vi "HEWH Assemble Test Sequence.vi"(8 "Error In":errorcluster, 11 "Cluster":T1 {"Time" format="%<%H:%M:%S>t"}) -> (0 "Error Out":errorcluster, 3 "String Test Seq":string[][](array[string]))   [LabVIEW 2016]
uses:
  Type Definitions/PRAT Test.ctl
  Utility/Save File/File Setup (Public)/Type Definition/Save File HEWH Heating Control Mode.ctl
  Draw Water Specific/Type Definitions/Terminate Draw Conditions.ctl
  Type Definitions/HEWH Start Conditions.ctl
  Draw Water Specific/Type Definitions/Check Special Condtions.ctl
  Draw Water Specific/Type Definitions/HEWH Special Condition Check.ctl
  Type Definitions/HEWH Draw Flag ENUM.ctl
  Utility/Save File/File Setup.lvlib
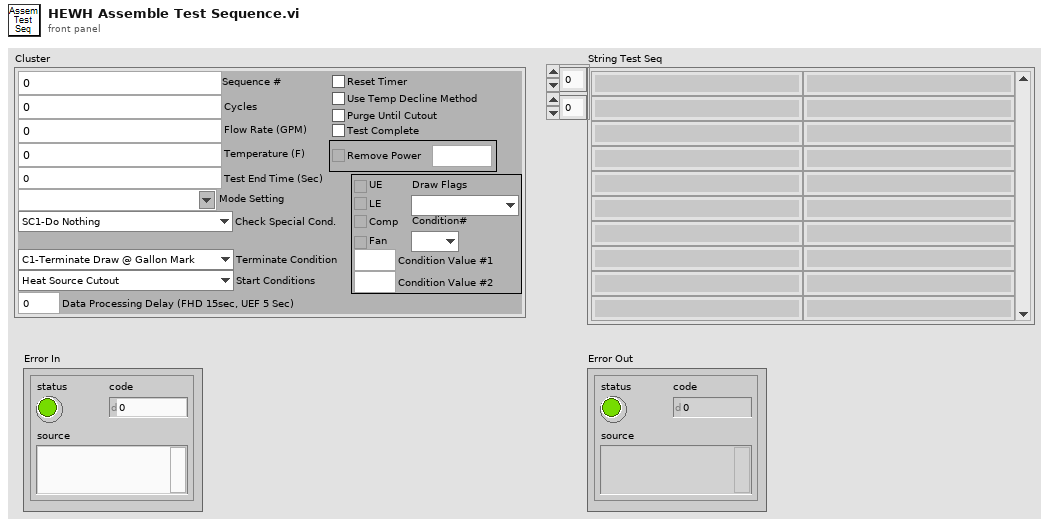
[diagram p1: front panel]
types:
  T1 = typedef "PRAT Test.ctl" = cluster{"Sequence #":dbl, "Cycles":i32, "Mode Setting":T2, "Flow Rate (GPM)":dbl, "Temperature (F)":dbl, "Reset Timer":bool, "Use Temp Decline Method":bool, "Terminate Condition":T3, "Condition Value #1":dbl, "UE":bool, "LE":bool, "Comp":bool, "Fan":bool, "Test End Time (Sec)":dbl, "Purge Until Cutout":bool, "Start Conditions":T4, "Condition Value #2":dbl, "Remove Power":bool, "Time":dbl, "Check Special Cond.":T5, "Condition#":T6, "Draw Flags":T7, "Data Processing Delay (FHD 15sec, UEF 5 Sec)":dbl, "Test Complete":bool}
  T2 = typedef "File Setup.lvlib/Save File HEWH Heating Control Mode.ctl" = string
  T3 = typedef "Terminate Draw Conditions.ctl" = enum16{"C1-Terminate Draw @ Gallon Mark", "C2-Special Last Draw (HU Test)", "C3-RTD Out <=", "C4-Mean Tank Temp <=", "C5-Decrease RTD Out (Deg F)", "C6-Time (Seconds)", "C7-Until Any Heat Source", "C8-Specific Heat Source", "C9-Do Nothing"}
  T4 = typedef "HEWH Start Conditions.ctl" = enum16{"Heat Source Cutout", "At Time (Seconds)", "Every X (Seconds)", "T2 >= X° Below Setpoint", "Seconds From Complete", "Wait for LE & Comp Cutout", "Wait for Comp Cutout", "Wait for LE Cutout", "Wait for UE Cutout"}
  T5 = typedef "Check Special Condtions.ctl" = enum16{"SC1-Do Nothing", "SC2-Check Heat Source (On-C2/Off-C1)", "SC3-Check Skip Condition", "SC4-Check Heat Source ON/Fail"}
  T6 = typedef "HEWH Special Condition Check.ctl" = enum16{"N/A", "C1", "C2", "Reset/Fail", "Skip Draw Sequence"}
  T7 = typedef "HEWH Draw Flag ENUM.ctl" = enum16{"N/A", "None(0)", "Sml(1)", "Med(2)", "SmlMed(3)", "Lrg(4)", "SmlLrg(5)", "MedLrg(6)", "SmlMedLrg(7)"}
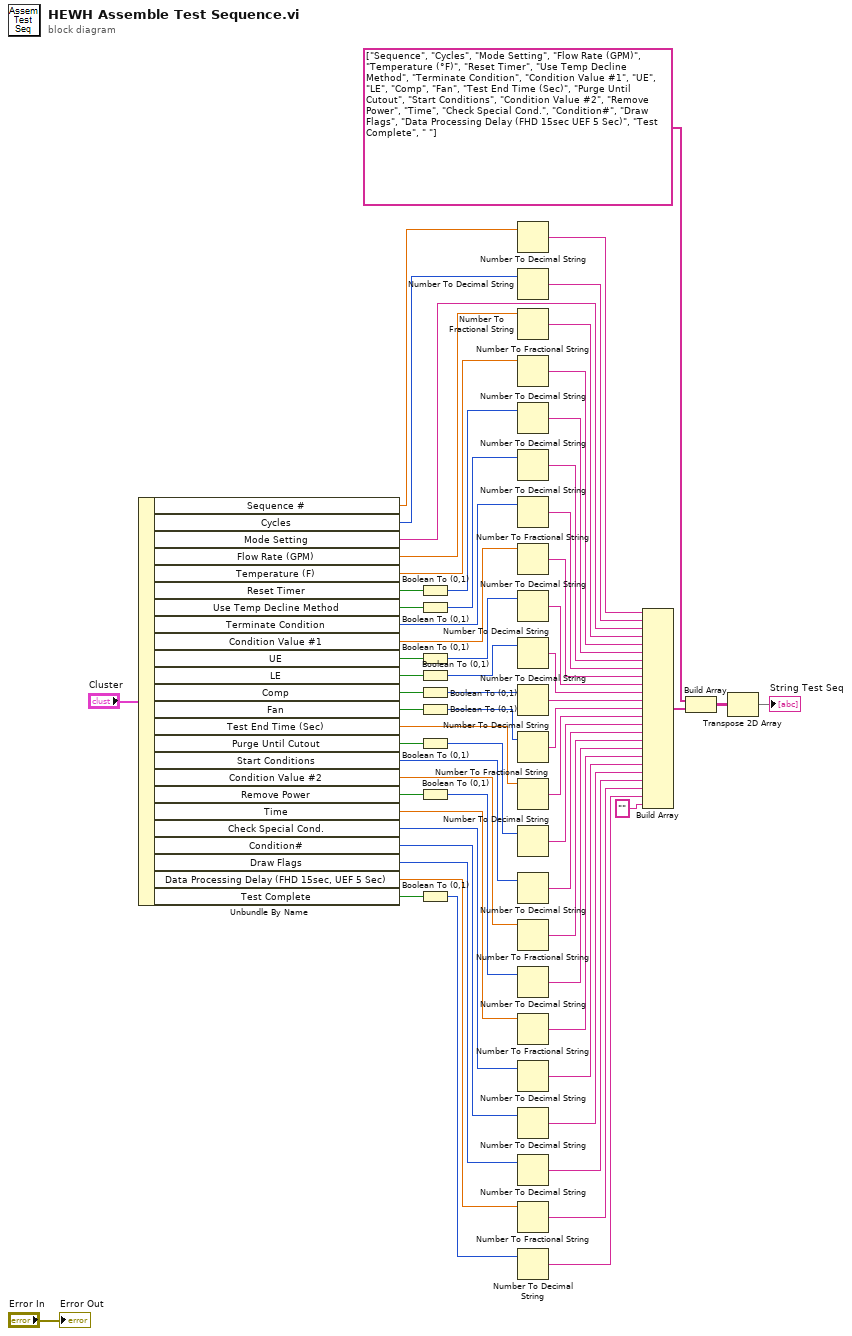
[diagram p0: block diagram]
diagram:
  n1 = Unbundle By Name("Cluster") -> ("Sequence #"=w3:dbl, "Cycles"=w9:i32, "Mode Setting"=w1:T2, "Flow Rate (GPM)"=w10:dbl, "Temperature (F)"=w11:dbl, "Reset Timer"=w12:bool, "Use Temp Decline Method"=w15:bool, "Terminate Condition"=w16:T3, "Condition Value #1"=w17:dbl, "UE"=w19:bool, "LE"=w21:bool, "Comp"=w23:bool, "Fan"=w25:bool, "Test End Time (Sec)"=w26:dbl, "Purge Until Cutout"=w28:bool, "Start Conditions"=w29:T4, "Condition Value #2"=w30:dbl, "Remove Power"=w32:bool, "Time"=w33:dbl, "Check Special Cond."=w34:T5, "Condition#"=w35:T6, "Draw Flags"=w36:T7, "Data Processing Delay (FHD 15sec, UEF 5 Sec)"=w37:dbl, "Test Complete"=w39:bool)
  n2 = Boolean To (0,1)(Boolean=w12) -> (0, 1=w13:i16)
  n3 = Boolean To (0,1)(Boolean=w15) -> (0, 1=w14:i16)
  n4 = Boolean To (0,1)(Boolean=w19) -> (0, 1=w18:i16)
  n5 = Boolean To (0,1)(Boolean=w21) -> (0, 1=w20:i16)
  n6 = Boolean To (0,1)(Boolean=w23) -> (0, 1=w22:i16)
  n7 = Boolean To (0,1)(Boolean=w25) -> (0, 1=w24:i16)
  n8 = Boolean To (0,1)(Boolean=w28) -> (0, 1=w27:i16)
  n9 = Boolean To (0,1)(Boolean=w32) -> (0, 1=w31:i16)
  n10 = Boolean To (0,1)(Boolean=w39) -> (0, 1=w38:i16)
  n11 = Number To Decimal String(number=w3) -> (decimal integer string=w2:string)  [unwired: 1 in]
  n12 = Number To Decimal String(number=w9) -> (decimal integer string=w40:string)  [unwired: 1 in]
  n13 = Number To Fractional String(number=w10) -> (F-format string=w41:string)  [unwired: 3 in]
  n14 = Number To Fractional String(number=w11) -> (F-format string=w42:string)  [unwired: 3 in]
  n15 = Number To Decimal String(number=w13) -> (decimal integer string=w43:string)  [unwired: 1 in]
  n16 = Number To Decimal String(number=w14) -> (decimal integer string=w44:string)  [unwired: 1 in]
  n17 = Number To Decimal String(number=w16) -> (decimal integer string=w45:string)  [unwired: 1 in]
  n18 = Number To Fractional String(number=w17) -> (F-format string=w46:string)  [unwired: 3 in]
  n19 = Number To Decimal String(number=w18) -> (decimal integer string=w47:string)  [unwired: 1 in]
  n20 = Number To Decimal String(number=w20) -> (decimal integer string=w48:string)  [unwired: 1 in]
  n21 = Number To Decimal String(number=w22) -> (decimal integer string=w49:string)  [unwired: 1 in]
  n22 = Number To Decimal String(number=w24) -> (decimal integer string=w50:string)  [unwired: 1 in]
  n23 = Number To Fractional String(number=w26) -> (F-format string=w51:string)  [unwired: 3 in]
  n24 = Number To Decimal String(number=w27) -> (decimal integer string=w52:string)  [unwired: 1 in]
  n25 = Number To Decimal String(number=w29) -> (decimal integer string=w53:string)  [unwired: 1 in]
  n26 = Number To Fractional String(number=w30) -> (F-format string=w54:string)  [unwired: 3 in]
  n27 = Number To Decimal String(number=w31) -> (decimal integer string=w55:string)  [unwired: 1 in]
  n28 = Number To Fractional String(number=w33) -> (F-format string=w56:string)  [unwired: 3 in]
  n29 = Number To Decimal String(number=w34) -> (decimal integer string=w57:string)  [unwired: 1 in]
  n30 = Number To Decimal String(number=w35) -> (decimal integer string=w58:string)  [unwired: 1 in]
  n31 = Number To Decimal String(number=w36) -> (decimal integer string=w59:string)  [unwired: 1 in]
  n32 = Number To Fractional String(number=w37) -> (F-format string=w60:string)  [unwired: 3 in]
  n33 = Number To Decimal String(number=w38) -> (decimal integer string=w61:string)  [unwired: 1 in]
  n34 = Build Array(w2, w40, w1, w41, w42, w43, w44, w45, w46, w47, w48, w49, w50, w51, w52, w53, w54, w55, w56, w57, w58, w59, w60, w61, "") -> (w63:T2[])
  n35 = Build Array(string[] ["Sequence", "Cycles", "Mode Setting", "Flow Rate (GPM)", "Temperature (°F)", "Reset Timer", "Use Temp Decline Method", "Terminate Condition", "Condition Value #1", "UE", "LE", "Comp", "Fan", "Test End Time (Sec)", "Purge Until Cutout", "Start Conditions", "Condition Value #2", "Remove Power", "Time", "Check Special Cond.", "Condition#", "Draw Flags", "Data Processing Delay (FHD 15sec UEF 5 Sec)", "Test Complete", " "], w63) -> (w6:T2[][])
  n36 = Transpose 2D Array(2D array=w6) -> (transposed array=→"String Test Seq":T2[][])
  "Error Out" <- "Error In"
